vi "Get Status.vi"(8 "error in (no error)":errorcluster, 11 "Command in":refnum<class "Command.lvclass">) -> (0 "error out":errorcluster, 2 "Status":string, 3 "Command out":refnum<class "Command.lvclass">)   [LabVIEW 2013, in "Command.lvclass"]
uses:
  Command.lvclass
  Command.lvclass/Command.ctl
  States/State/State.lvclass
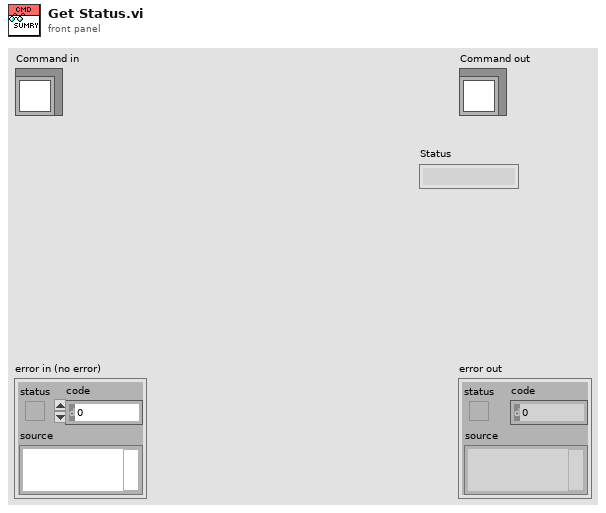
[diagram p1: front panel]
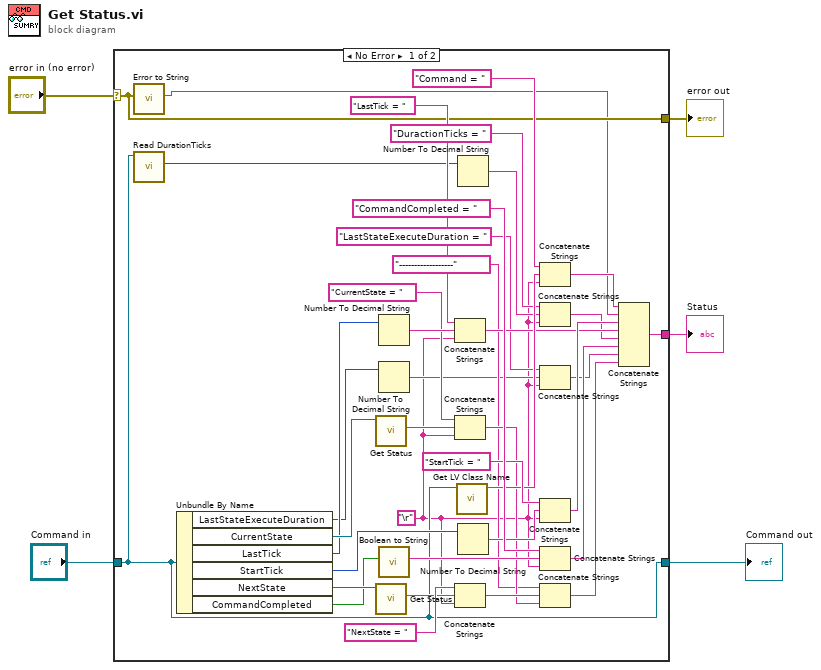
[diagram p0: block diagram]
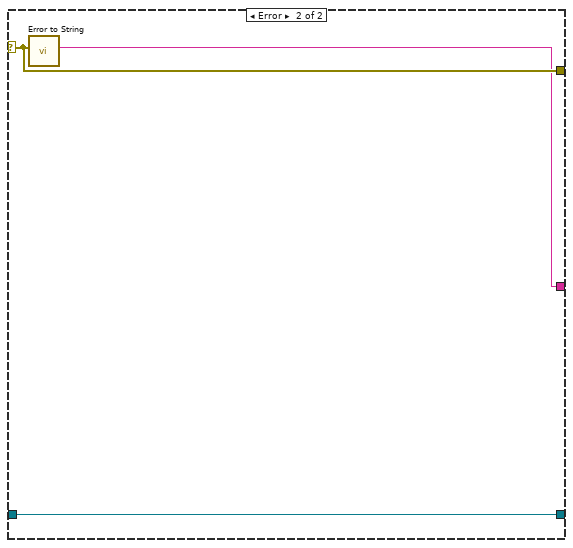
[diagram p2: hidden frame]
diagram:
  n1 = case shown="No Error" "error in (no error)" {
    selector: "error in (no error)" -> [w33 w45]
    tunnel: [w33 w45] -> w4
    tunnel: [w23 w46] -> w2
    tunnel: "Command in" -> [w23 w46]
    tunnel: [w15 w44] -> w1
    frame No Error {
      w6 = "\r"
      n2 = call "Error to String.vi"("error in (no error)"=w33) -> ("String out"=w20:string)  [unwired: 10 in]
      n3 = call-dynamic "Read DurationTicks.vi"("Command in"=w23) -> ("DurationTicks"=w22:u32)  [unwired: 8 in, 2 out]
      n4 = Unbundle By Name(w23) -> ("LastStateExecuteDuration"=w8:u32, "CurrentState"=w30:refnum<class "State.lvclass">, "LastTick"=w24:u32, "StartTick"=w43:u32, "NextState"=w32:refnum<class "State.lvclass">, "CommandCompleted"=w28:bool)
      n5 = call-dynamic "Get Status.vi"("State in"=w30) -> ("Status"=w29:string)  [unwired: 8 in, 2 out]
      n6 = call-dynamic "Get Status.vi"("State in"=w32) -> ("Status"=w31:string)  [unwired: 8 in, 2 out]
      n7 = Number To Decimal String(number=w24) -> (decimal integer string=w38:string)  [unwired: 1 in]
      n8 = Number To Decimal String(number=w8) -> (decimal integer string=w7:string)  [unwired: 1 in]
      n9 = call "Boolean to String.vi"("Boolean"=w28) -> ("String"=w27:string)  [unwired: 10 in]
      n10 = Concatenate Strings("LastTick = ", w38, w6) -> (w18:string)
      n11 = Concatenate Strings("CurrentState = ", w29, w6) -> (w11:string)
      n12 = Concatenate Strings("NextState = ", w31, w6) -> (w12:string)
      n13 = call <vilib>:"Get LV Class Name.vi"("object"=w23) -> ("class name"=w34:string)  [unwired: 9 in, 1 out]
      n14 = Number To Decimal String(number=w22) -> (decimal integer string=w25:string)  [unwired: 1 in]
      n15 = Number To Decimal String(number=w43) -> (decimal integer string=w40:string)  [unwired: 1 in]
      n16 = Concatenate Strings("Command = ", w34, w6) -> (w21:string)
      n17 = Concatenate Strings("DuractionTicks = ", w25, w6) -> (w17:string)
      n18 = Concatenate Strings("LastStateExecuteDuration = ", w7, w6) -> (w13:string)
      n19 = Concatenate Strings("StartTick = ", w40, w6) -> (w19:string)
      n20 = Concatenate Strings("CommandCompleted = ", w27, w6) -> (w16:string)
      n21 = Concatenate Strings("------------------", w12, w11) -> (w9:string)
      n22 = Concatenate Strings(w21, w20, w19, w18, w17, w16, w13, w9) -> (w15:string)
    }
    frame Error {
      n23 = call "Error to String.vi"("error in (no error)"=w45) -> ("String out"=w44:string)  [unwired: 10 in]
    }
  }
  "error out" <- w4
  "Command out" <- w2
  "Status" <- w1
